vi "Test_logEvent_logMessage.vi"(8 "error in (no error)":errorcluster, 11 "logevent_logMessage_Ctl":T1) -> (0 "error out":errorcluster, 2 "function return":i32, 3 "logevent_logMessage_Ctl out":T1)   [LabVIEW 2018, in "SALLV_Test.lvlib"]
doc: "int Test_shm_logEvent_logMessageLV(Test_logevent_logMessageLV *logevent_logMessage_Ctl );"
uses:
  DataTypes/logevent_logMessage.ctl
  SALLV_Test.lvlib
  SALLV_Test.so
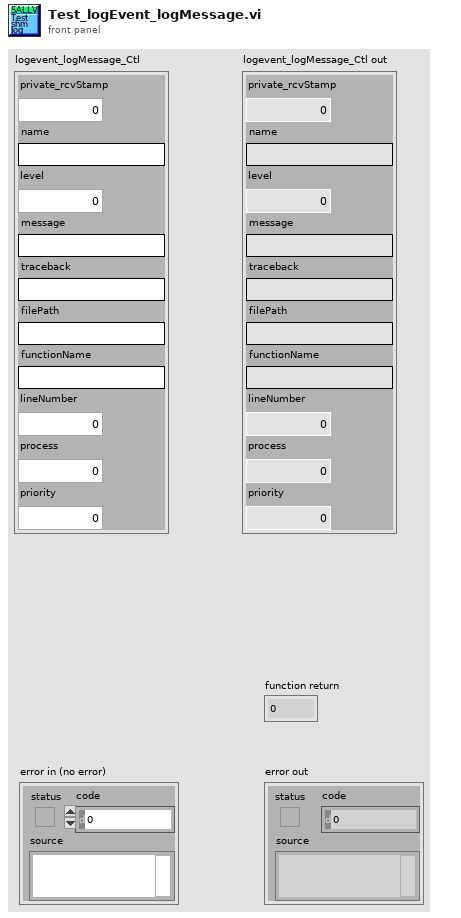
[diagram p1: front panel]
types:
  T1 = typedef "SALLV_Test.lvlib/logevent_logMessage.ctl" = cluster{"private_rcvStamp":dbl, "name":string, "level":i32, "message":string, "traceback":string, "filePath":string, "functionName":string, "lineNumber":i32, "process":i32, "priority":i32}
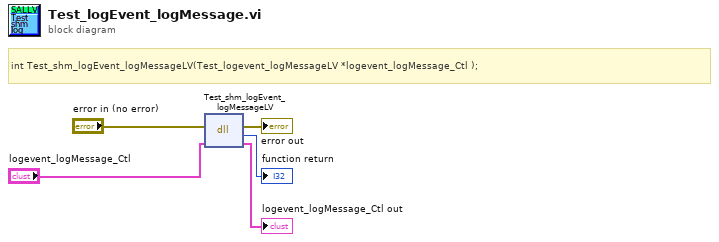
[diagram p0: block diagram]
diagram:
  # "int Test_shm_logEvent_logMessageLV(Test_logevent_logMessageLV *logevent_logMessage_Ctl );"
  n1 = dll-call lib="home/ttsai/Documents/salTestLabViewApi/SALLV_Test/SALLV_Test.*" fn="Test_shm_logEvent_logMessageLV"(error in="error in (no error)", "logevent_logMessage_Ctl"="logevent_logMessage_Ctl") -> (error out=→"error out":errorcluster, →"function return":i32, "logevent_logMessage_Ctl"=→"logevent_logMessage_Ctl out":T1)  [unwired: 2 in, 1 out]
